vi "Track Blocks.vi"(8 "Url":string="169.254.66.20:8080/shot.jpg", 9 "client handle":T1=refnum, 10 "Image Dst":T2=refnum, 11 "New Image":T2=refnum) -> (1 "Object found?":bool=TRUE, 2 "Object Output":cluster{"X":i32, "Y":i32}={"X"=189, "Y"=422}, 3 "Image Out":T2)   [LabVIEW 2012]
uses:
  <vilib>/vision/Image Controls.llb/IMAQ Image.ctl
  <vilib>/httpClient/ClientHandle.ctl
  <vilib>/httpClient/LabVIEWHTTPClient.lvlib
panel:
  in  "Area Lower Limit":dbl=2000.0
  in  "Area Upper Limit":dbl=70000.0
  out "Blob Area":dbl=25411.0
  in  "Show Image":bool
  out "Camera":T2(plugin-control)
  out "Particle Measurements (Pixels)":dbl[][](array[numeric])=[[1.0, 122.0, 123.0, 142.0, 143.0, 142.0, 122.0], [10.0, 125.0, 127.0, 136.0, 144.0, 140.1, 125.8], [1.0, 126.0, 127.0, 289.0, 290.0, 289.0, 126.0], [1.0, 133.0, 134.0, 103.0, 104.0, 103.0, 133.0], [7.0, 145.0, 147.0, 94.0, 100.0, 96.71428571428571, 145.28571428571428], [2.0, 145.0, 146.0, 102.0, 104.0, 102.5, 145.0], [18.0, 145.0, 151.0, 104.0, 111.0, 107.66666666666667, 147.22222222222223], [3.0, 154.0, 155.0, 124.0, 127.0, 125.0, 154.0], [2.0, 154.0, 155.0, 145.0, 147.0, 145.5, 154.0], [25.0, 162.0, 166.0, 113.0, 127.0, 120.56, 163.72], [1.0, 165.0, 166.0, 111.0, 112.0, 111.0, 165.0], [17.0, 169.0, 172.0, 87.0, 96.0, 91.47058823529412, 170.11764705882354], [1.0, 172.0, 173.0, 84.0, 85.0, 84.0, 172.0], [4.0, 174.0, 175.0, 75.0, 79.0, 76.5, 174.0], [38.0, 177.0, 182.0, 49.0, 64.0, 57.28947368421053, 179.42105263157896], [2.0, 193.0, 194.0, 270.0, 272.0, 270.5, 193.0], [34.0, 202.0, 207.0, 69.0, 80.0, 75.11764705882354, 203.5], [14.0, 209.0, 214.0, 86.0, 95.0, 90.14285714285714, 210.78571428571428], [2.0, 209.0, 211.0, 94.0, 95.0, 94.0, 209.5], [1.0, 216.0, 217.0, 131.0, 132.0, 131.0, 216.0], [10.0, 218.0, 221.0, 106.0, 112.0, 108.8, 218.7], [28.0, 226.0, 231.0, 101.0, 112.0, 106.78571428571429, 228.17857142857142], [1.0, 230.0, 231.0, 99.0, 100.0, 99.0, 230.0], [10.0, 231.0, 234.0, 91.0, 96.0, 93.1, 231.9], [1.0, 234.0, 235.0, 87.0, 88.0, 87.0, 234.0], [11.0, 236.0, 239.0, 73.0, 80.0, 76.54545454545455, 237.45454545454547], [3.0, 238.0, 239.0, 144.0, 147.0, 145.0, 238.0], [32.0, 242.0, 247.0, 53.0, 64.0, 59.125, 244.125], [7.0, 244.0, 248.0, 161.0, 166.0, 162.85714285714286, 245.28571428571428], [20.0, 247.0, 251.0, 40.0, 48.0, 44.35, 248.7], [8.0, 253.0, 256.0, 25.0, 31.0, 27.75, 254.25], [5.0, 254.0, 256.0, 43.0, 48.0, 45.0, 254.6], [1.0, 254.0, 255.0, 184.0, 185.0, 184.0, 254.0], [1.0, 254.0, 255.0, 319.0, 320.0, 319.0, 254.0], [1.0, 255.0, 256.0, 33.0, 34.0, 33.0, 255.0], [1.0, 255.0, 256.0, 317.0, 318.0, 317.0, 255.0], [6.0, 258.0, 260.0, 194.0, 198.0, 195.16666666666666, 258.6666666666667], [18.0, 259.0, 264.0, 6.0, 16.0, 11.61111111111111, 260.72222222222223], [1.0, 260.0, 261.0, 192.0, 193.0, 192.0, 260.0], [1.0, 263.0, 264.0, 3.0, 4.0, 3.0, 263.0], [1.0, 263.0, 264.0, 11.0, 12.0, 11.0, 263.0], [2.0, 263.0, 265.0, 302.0, 304.0, 302.5, 263.5], [2.0, 266.0, 268.0, 298.0, 300.0, 298.5, 266.5], [6.0, 268.0, 271.0, 293.0, 297.0, 294.5, 269.0], [6.0, 268.0, 271.0, 317.0, 320.0, 318.3333333333333, 269.3333333333333], [1.0, 271.0, 272.0, 227.0, 228.0, 227.0, 271.0], [2.0, 271.0, 272.0, 288.0, 290.0, 288.5, 271.0], [1.0, 271.0, 272.0, 293.0, 294.0, 293.0, 271.0], [1.0, 271.0, 272.0, 299.0, 300.0, 299.0, 271.0], [9.0, 273.0, 276.0, 282.0, 288.0, 284.44444444444446, 274.1111111111111], [1.0, 276.0, 277.0, 240.0, 241.0, 240.0, 276.0], [4.0, 276.0, 278.0, 278.0, 281.0, 279.0, 276.75], [3.0, 276.0, 278.0, 285.0, 288.0, 286.0, 276.6666666666667], [2.0, 277.0, 278.0, 243.0, 245.0, 243.5, 277.0], [4.0, 282.0, 284.0, 269.0, 271.0, 269.5, 282.5], [2.0, 289.0, 290.0, 242.0, 244.0, 242.5, 289.0], [15.0, 304.0, 307.0, 217.0, 224.0, 220.26666666666668, 304.93333333333334], [1.0, 304.0, 305.0, 225.0, 226.0, 225.0, 304.0], [1.0, 307.0, 308.0, 209.0, 210.0, 209.0, 307.0], [8.0, 309.0, 312.0, 208.0, 213.0, 210.0, 310.125], [19.0, 320.0, 326.0, 176.0, 180.0, 177.6315789473684, 322.6842105263158], [30.0, 320.0, 324.0, 186.0, 198.0, 191.03333333333333, 321.03333333333336], [14.0, 322.0, 328.0, 204.0, 208.0, 205.85714285714286, 324.2142857142857], [10.0, 327.0, 331.0, 180.0, 186.0, 182.1, 328.3], [25411.0, 327.0, 480.0, 36.0, 320.0, 188.71976703002636, 421.7554208807209], [3.0, 328.0, 330.0, 177.0, 179.0, 177.33333333333334, 328.3333333333333], [1.0, 332.0, 333.0, 176.0, 177.0, 176.0, 332.0], [33.0, 336.0, 343.0, 155.0, 166.0, 159.3030303030303, 338.3333333333333], [1.0, 338.0, 339.0, 167.0, 168.0, 167.0, 338.0], [1.0, 340.0, 341.0, 237.0, 238.0, 237.0, 340.0], [16.0, 346.0, 351.0, 144.0, 149.0, 145.8125, 348.5], [1.0, 352.0, 353.0, 5.0, 6.0, 5.0, 352.0], [2.0, 352.0, 354.0, 7.0, 8.0, 7.0, 352.5], [1.0, 352.0, 353.0, 9.0, 10.0, 9.0, 352.0], [1.0, 352.0, 353.0, 11.0, 12.0, 11.0, 352.0], [31.0, 352.0, 368.0, 259.0, 262.0, 260.0, 359.741935483871], [13.0, 355.0, 360.0, 264.0, 269.0, 265.6923076923077, 357.15384615384613], [111.0, 355.0, 369.0, 271.0, 282.0, 274.9189189189189, 362.22522522522524], [4.0, 356.0, 358.0, 10.0, 12.0, 10.5, 356.5], [6.0, 357.0, 362.0, 14.0, 16.0, 14.833333333333334, 359.1666666666667], [1.0, 368.0, 369.0, 23.0, 24.0, 23.0, 368.0], [28.0, 368.0, 374.0, 96.0, 103.0, 98.64285714285714, 369.64285714285717], [23.0, 369.0, 377.0, 25.0, 32.0, 28.652173913043477, 372.4782608695652], [1.0, 369.0, 370.0, 31.0, 32.0, 31.0, 369.0], [4.0, 369.0, 372.0, 126.0, 128.0, 126.75, 370.0], [3.0, 370.0, 372.0, 120.0, 122.0, 120.33333333333333, 370.3333333333333], [11.0, 374.0, 379.0, 141.0, 147.0, 143.45454545454547, 375.72727272727275], [3.0, 376.0, 377.0, 133.0, 136.0, 134.0, 376.0], [29.0, 382.0, 387.0, 264.0, 272.0, 268.3103448275862, 383.58620689655174], [22.0, 384.0, 392.0, 41.0, 48.0, 44.59090909090909, 386.6818181818182], [92.0, 384.0, 390.0, 64.0, 80.0, 71.34782608695652, 386.44565217391306], [5.0, 384.0, 387.0, 299.0, 301.0, 299.4, 385.2], [5.0, 394.0, 397.0, 64.0, 67.0, 65.2, 395.0], [1.0, 400.0, 401.0, 57.0, 58.0, 57.0, 400.0], [92.0, 417.0, 432.0, 41.0, 52.0, 47.59782608695652, 426.14130434782606], [38.0, 425.0, 432.0, 21.0, 31.0, 26.5, 428.7631578947368], [6.0, 428.0, 431.0, 36.0, 39.0, 36.833333333333336, 429.0], [1.0, 431.0, 432.0, 19.0, 20.0, 19.0, 431.0], [1.0, 432.0, 433.0, 74.0, 75.0, 74.0, 432.0], [57.0, 433.0, 443.0, 5.0, 16.0, 11.771929824561404, 437.82456140350877], [1273.0, 444.0, 480.0, 0.0, 48.0, 19.72191673212883, 461.83896307934015]] format="%.2f"
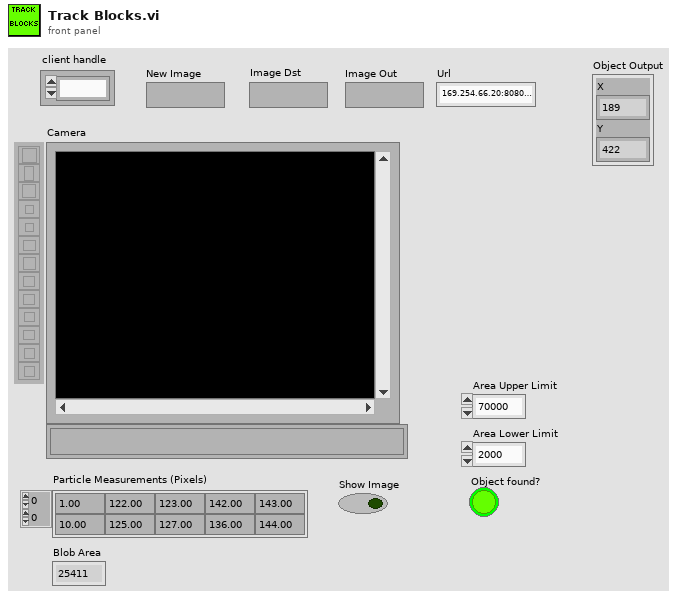
[diagram p1: front panel]
types:
  T1 = typedef "LabVIEWHTTPClient.lvlib/ClientHandle.ctl" = refnum<k1>
  T2 = typedef "IMAQ Image.ctl" = refnum<image>
  T3 = cluster{"X Velocity (m/s)":dbl, "Y Velocity (m/s)":dbl, "Angular Velocity (rad/s)":dbl}
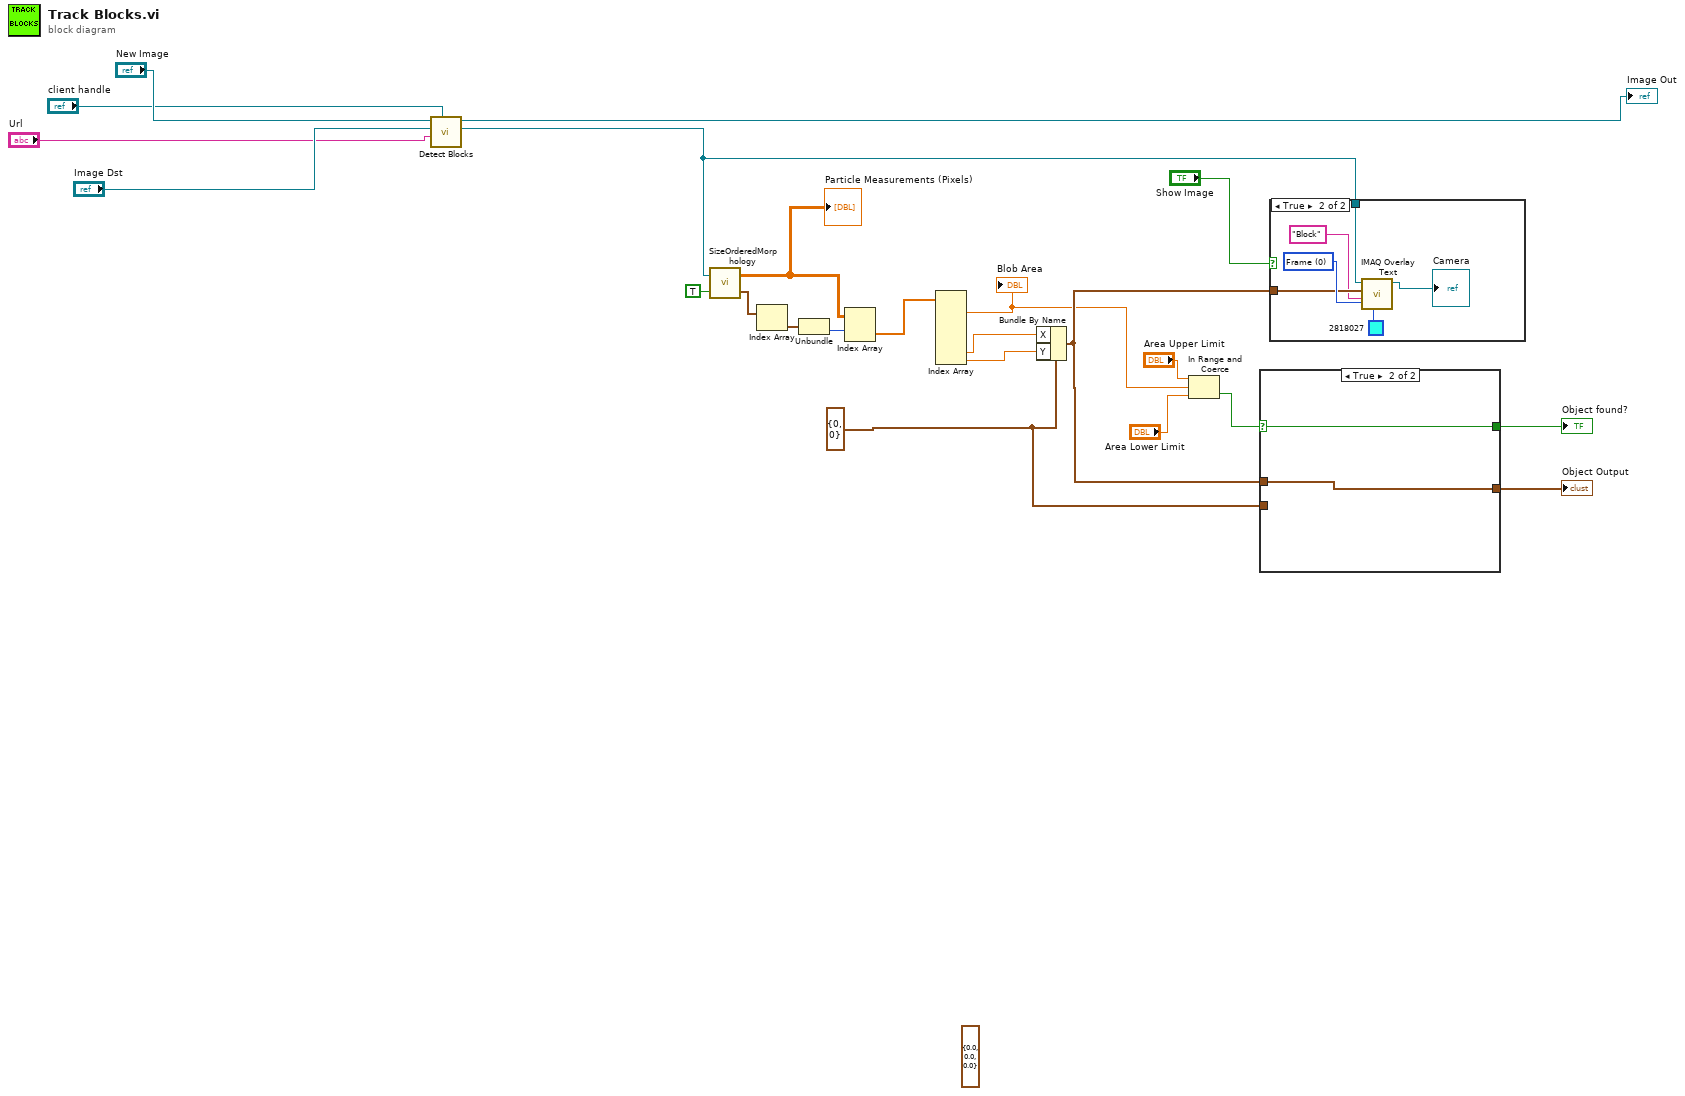
[diagram p0: block diagram]
diagram:
  (unwired) T3 {"X Velocity (m/s)"=0.0, "Y Velocity (m/s)"=0.0, "Angular Velocity (rad/s)"=0.0} ("Robot Velocities")
  w8 = cluster{"X":i32, "Y":i32} {"X"=0, "Y"=0} ("Origin")
  n1 = call "Detect Blocks.vi"("client handle"="client handle", "Url"="Url", "Image Dst"="Image Dst", "Refnum in"="New Image") -> ("Detected Image Out"=w13:T2, "Camer Image out"=→"Image Out":T2)  [unwired: 5 in, 1 out]
  n2 = call "SizeOrderedMorphology.vi"("Green"=TRUE, "Image Dst Out"=w13) -> ("Sort Array"=w20:cluster{"Numeric":dbl, i32}[], "Particle Measurements (Pixels)"=w16:dbl[][])
  "Particle Measurements (Pixels)" <- w16
  n3 = Index Array(array=w20) -> (element=w19:cluster{"Numeric":dbl, i32})  [unwired: 1 in]
  n4 = Unbundle(w19) -> (w18:i32)  [unwired: 1 out]
  n5 = Index Array(array=w16, index (row)=w18) -> (element=w17:dbl[])  [unwired: 1 in]
  n6 = Index Array(array=w17) -> (element #1=w6:dbl, element #6=w14:dbl, element #7=w15:dbl)  [unwired: 7 in, 4 out]
  "Blob Area" <- w6
  n7 = Bundle By Name(cluster=w8, "X"=w14, "Y"=w15) -> (w22:cluster{"X":i32, "Y":i32})
  n8 = In Range and Coerce(upper limit="Area Upper Limit", x=w6, lower limit="Area Lower Limit") -> (In Range?=w7:bool)  [unwired: 1 out]
  n9 = case shown="True" w7 {
    selector: w7 -> [w24 w26]
    tunnel: w22 -> [_ w27]
    tunnel: [w25 w27] -> w9
    tunnel: w8 -> [w25 _]
    tunnel: [w24 w26] -> w3
    frame False {
    }
    frame True {
    }
  }
  "Object Output" <- w9
  "Object found?" <- w3
  n10 = case shown="True" "Show Image" {
    tunnel: w22 -> [_ w31]
    tunnel: w13 -> [_ w28]
    frame False {
    }
    frame True {
      w32 = u32 0 items=["Frame", "Fill", "Highlight"] ("Drawing Mode (Frame)")
      n11 = call "IMAQ Overlay Text"("BG Color (Transparent)"=w32, "Text Color (black)"=u32 2818027 ("Color"), "String"="Block", "Origin"=w31, "Image"=w28) -> ("Image Out"=→"Camera":T2)  [unwired: 5 in, 1 out]
    }
  }
